vi "util_gen_cmd_error.vi"(6 "ignore_code":bool, 8 "error in (no error)":errorcluster, 10 "return_code":i32, 11 "standard_error":string) -> (0 "error out":errorcluster)   [LabVIEW 2015, in "lv-bin.lvlib" / "v1.lvlib"]
uses:
  v1.lvlib
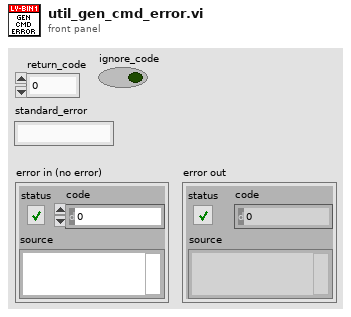
[diagram p1: front panel]
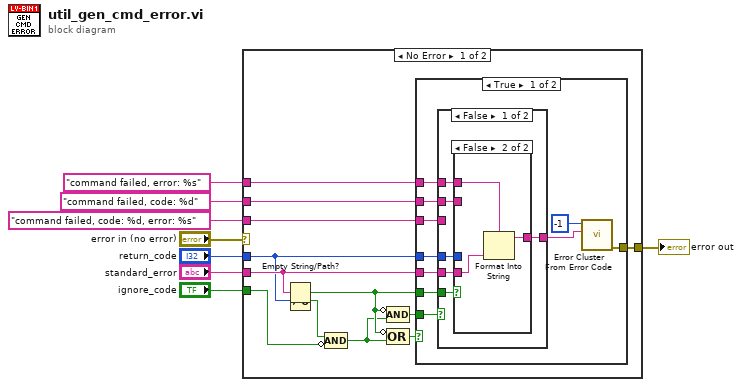
[diagram p0: block diagram]
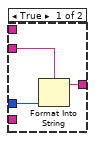
[diagram p2: hidden frame]
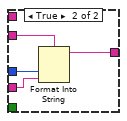
[diagram p3: hidden frame]
diagram:
  n1 = case shown="No Error" "error in (no error)" {
    selector: "error in (no error)" -> [_ w47]
    tunnel: [w19 w47] -> w7
    tunnel: "standard_error" -> [w18 _]
    tunnel: "command failed, error: %s" ("format string") -> [w20 _]
    tunnel: "return_code" -> [w15 _]
    tunnel: "command failed, code: %d" ("format string") -> [w14 _]
    tunnel: "command failed, code: %d, error: %s" ("format string") -> [w13 _]
    tunnel: "ignore_code" -> [w11 _]
    frame No Error {
      n2 = Empty String/Path?(string/path=w18) -> (empty?=w12:bool)
      n3 = Not Equal To 0?(x=w15) -> (x != 0?=w10:bool)
      n4 = Compound Arithmetic op=AND(w10, invert w11) -> (w9:bool)
      n5 = Compound Arithmetic op=AND(invert w12, w9) -> (w16:bool)
      n6 = Compound Arithmetic op=OR(invert w12, w9) -> (w17:bool)
      n7 = case shown="True" w17 {
        tunnel: w20 -> [w30 _]
        tunnel: [w29 _] -> w19
        tunnel: w12 -> [w24 _]
        tunnel: w16 -> [w25 _]
        tunnel: w15 -> [w23 _]
        tunnel: w18 -> [w26 _]
        tunnel: w14 -> [w21 _]
        tunnel: w13 -> [w22 _]
        frame True {
          n8 = case shown="False" w25 {
            tunnel: w30 -> [w36 _]
            tunnel: [w35 w46] -> w28
            tunnel: w26 -> [w34 w43]
            tunnel: w24 -> [w33 _]
            tunnel: w23 -> [w31 w44]
            tunnel: w22 -> [_ w45]
            tunnel: w21 -> [w32 _]
            frame False {
              n9 = case shown="False" w33 {
                tunnel: w36 -> [_ w41]
                tunnel: [w39 w42] -> w35
                tunnel: w34 -> [_ w40]
                tunnel: w32 -> [w38 _]
                tunnel: w31 -> [w37 _]
                frame True {
                  n10 = Format Into String(format string=w38, w37) -> (resulting string=w39:string)  [unwired: 2 in, 1 out]
                }
                frame False {
                  n11 = Format Into String(format string=w41, w40) -> (resulting string=w42:string)  [unwired: 2 in, 1 out]
                }
              }
            }
            frame True {
              n12 = Format Into String(format string=w45, w44, w43) -> (resulting string=w46:string)  [unwired: 2 in, 1 out]
            }
          }
          n13 = call <vilib>:"Error Cluster From Error Code.vi"("error message (\"\")"=w28, "error code (0)"=-1) -> ("error out"=w29:errorcluster)  [unwired: 7 in]
        }
        frame False {
        }
      }
    }
    frame Error {
    }
  }
  "error out" <- w7
